vi "Decoder.vi"() -> ()   [LabVIEW 2021]
panel:
  in  "B":bool
  in  "A":bool
  out "Q3":bool
  out "Q2":bool
  out "Q1":bool
  out "Q0":bool
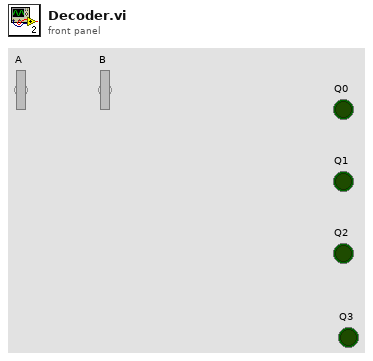
[diagram p1: front panel]
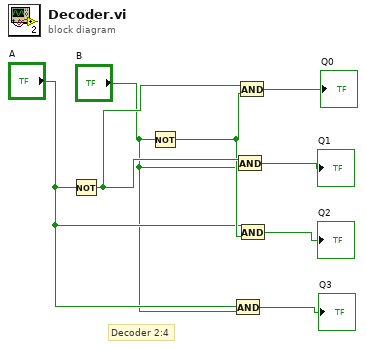
[diagram p0: block diagram]
diagram:
  # "Decoder 2:4"
  n1 = Not(x="A") -> (.not. x?=w4:bool)
  n2 = Not(x="B") -> (.not. x?=w3:bool)
  n3 = And(x="A", y="B") -> (x .and. y?=→"Q3":bool)
  n4 = And(x=w4, y="B") -> (x .and. y?=→"Q1":bool)
  n5 = And(x=w4, y=w3) -> (x .and. y?=→"Q0":bool)
  n6 = And(x="A", y=w3) -> (x .and. y?=→"Q2":bool)
